vi "SETPATHdll_Test.vi"(8 "error in (no error)":errorcluster) -> (0 "error out":errorcluster, 3 "Passed?":bool)   [LabVIEW 2016]
panel:
  out "hpath out":string
  out "ln":i32
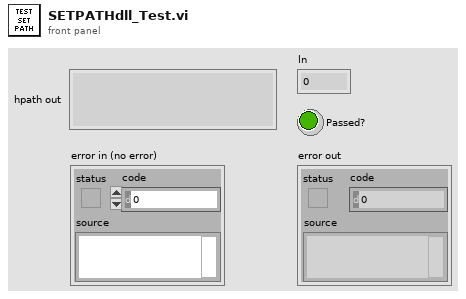
[diagram p1: front panel]
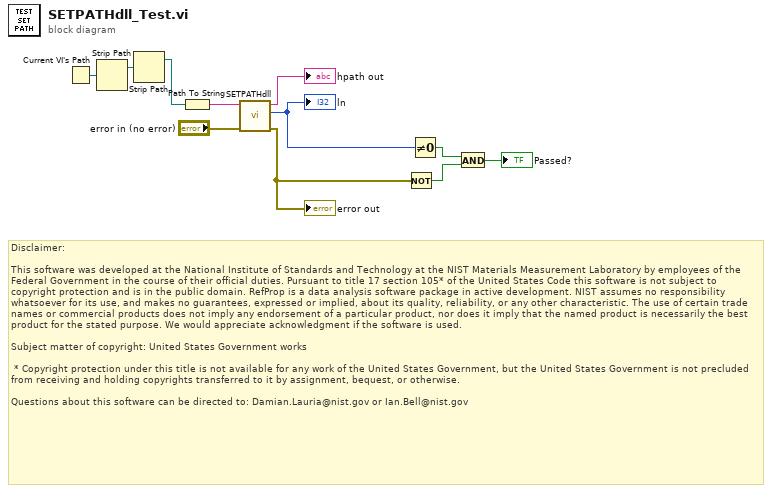
[diagram p0: block diagram]
diagram:
  # "Disclaimer:\n\nThis software was developed at the National Institute of Standards and Technology at the NIST Materials Measurement Laboratory by employees of the Federal Government in the course of their official duties. Pursuant to title 17 section 105* of the United States Code this software is not subject to copyright protection and is in the public domain. RefProp is a data analysis software package in active development. NIST assumes no responsibility whatsoever for its use, and makes no guarantees, expressed or implied, about its quality, reliability, or any other characteristic. The use of certain trade names or commercial products does not imply any endorsement of a particular product, nor does it imply that the named product is necessarily the best product for the stated purpose. We would appreciate acknowledgment if the software is used.\n \nSubject matter of copyright: United States Government works\n  \n * Copyright protection under this title is not available for any work of the United States Government, but the United States Government is not precluded from receiving and holding copyrights transferred to it by assignment, bequest, or otherwise.\n\nQuestions about this software can be directed to: Damian.Lauria@nist.gov or Ian.Bell@nist.gov"
  n1 = Current VI's Path() -> (path=w3:path)
  n2 = Strip Path(path=w3) -> (stripped path=w2:path)  [unwired: 1 out]
  n3 = Strip Path(path=w2) -> (stripped path=w1:path)  [unwired: 1 out]
  n4 = Path To String(path=w1) -> (string=w9:string)
  n5 = call "SETPATHdll.vi"("error in (no error)"="error in (no error)", "hpath"=w9) -> ("error out"=w7:errorcluster, "ln"=w8:i32, "hpath out"=→"hpath out":string)  [unwired: 7 in]
  "error out" <- w7
  "ln" <- w8
  n6 = Not(x=w7) -> (.not. x?=w5:bool)
  n7 = Not Equal To 0?(x=w8) -> (x != 0?=w6:bool)
  n8 = And(x=w6, y=w5) -> (x .and. y?=→"Passed?":bool)
